vi "Type Panel.vi"(11 "StringPanel in":refnum<class "StringPanel.lvclass">) -> ()   [LabVIEW 2020, in "Conditum-Tools.lvlib" / "StringPanel.lvclass"]
uses:
  StringPanel.lvclass
  C:/dev/lv20CE/lv-conditum-tools/Conditum-Tools/ColumnPanel/ColumnPanel.lvclass
  Conditum-Clone/Columns/String/String.lvclass
  ColumnPanel/ColumnPanel.lvclass
panel:
  in  "Length":i32=255
  in  "Default":string
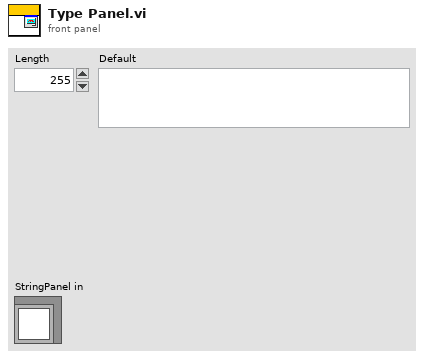
[diagram p1: front panel]
types:
  T1 = typedef "Conditum-Tools.lvlib/ColumnPanel.lvclass/Type Panel Event Reg.ctl" = refnum<event-registration>
  T2 = typedef "Conditu2.lvlib/Columns.lvlib/String.lvclass/Definition.ctl" = cluster{"Default":string, "Length":i32}
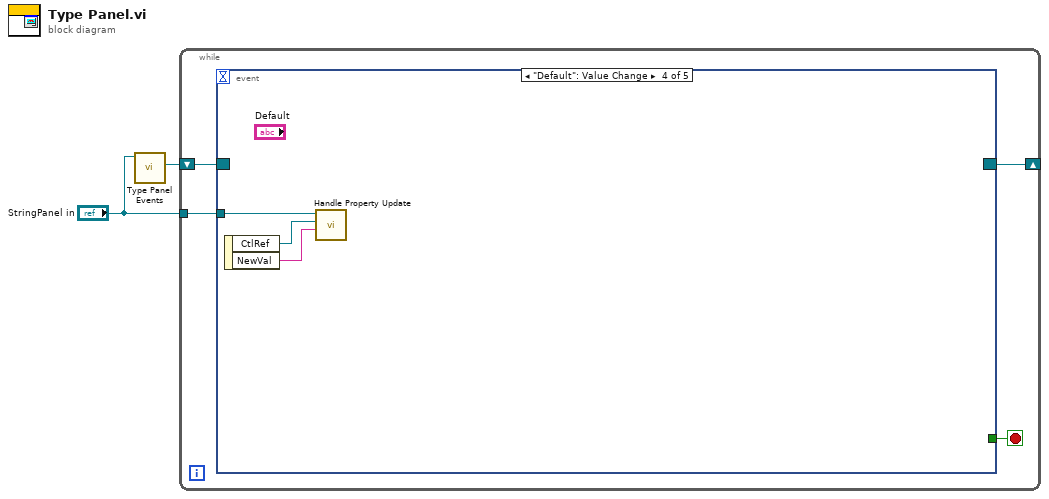
[diagram p0: block diagram]
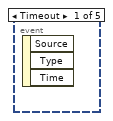
[diagram p2: hidden frame]
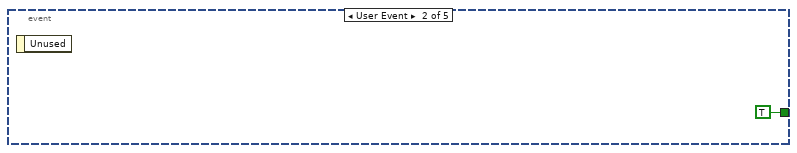
[diagram p3: hidden frame]
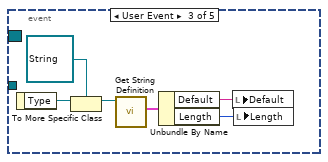
[diagram p4: hidden frame]
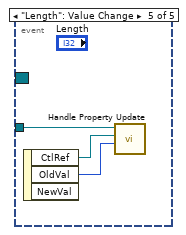
[diagram p5: hidden frame]
diagram:
  n1 = call "Type Panel Events.vi"("ColumnPanel"="StringPanel in") -> ("Type Panel Event Reg"=w2:T1)  [unwired: 10 in]
  n2 = while {
    tunnel: "StringPanel in" -> [w5]
    shift-right: [w3] -> _
    shift-left: w2 -> [w4]
    stop <- w6 stop-if-true
    n3 = event shown="[3] \"Default\": Value Change" {
      selector: w4 -> [_ _ _ _ _]
      dyn-events: [_ _ _ _ _] -> w3
      timeout: _ -> [_ _ _ _ _]
      tunnel: [_ TRUE _ _ _] -> w6
      tunnel: w5 -> [_ _ _ w16 w19]
      event Timeout {
        n4 = event-data() -> ()  [unwired: 1 in, 3 out]
      }
      event User Event {
        n5 = event-data() -> ()  [unwired: 1 in, 1 out]
      }
      event User Event {
        n6 = event-data() -> ("Type"=w13:refnum<class "Type.lvclass">)  [unwired: 1 in]
        n7 = To More Specific Class(target class=refnum<class "String.lvclass"> refnum ("Boolean"), reference=w13) -> (specific class reference=w10:refnum<class "String.lvclass">)  [unwired: 1 in, 1 out]
        n8 = call "Get String Definition.vi"("String in"=w10) -> ("Definition"=w9:T2)  [unwired: 10 in]
        n9 = Unbundle By Name(w9) -> ("Default"=w12:string, "Length"=w8:i32)
        n10 = local write "Default"(w12) -> ()
        n11 = local write "Length"(w8) -> ()
      }
      event "Default": Value Change {
        n12 = event-data() -> ("CtlRef"=w15:refnum<vi>, "NewVal"=w14:string)  [unwired: 1 in]
        n13 = call "Handle Property Update.vi"("Value"=w14, "Control"=w15, "ColumnPanel in"=w16) -> ()  [unwired: 7 in, 2 out]
      }
      event "Length": Value Change {
        n14 = event-data() -> ("CtlRef"=w18:refnum<vi>, "OldVal"=w17:i32)  [unwired: 1 in, 1 out]
        n15 = call "Handle Property Update.vi"("Value"=w17, "Control"=w18, "ColumnPanel in"=w19) -> ()  [unwired: 7 in, 2 out]
      }
    }
  }
